vi "CheckExportedFunctionCallCoverage.vi"() -> ()   [LabVIEW 2020]
uses:
  <vilib>/Utility/traverseref.llb/TRef TravTarget.ctl
  02b7a759-a23e-437a-9814-93bb2d072b00.vi
  <vilib>/Utility/traverseref.llb/VI Scripting - Traverse.lvlib
panel:
  out "In Source but not called by LabVIEW":set{string}(c389)
  out "Specified in C++ Source":set{string}(c389)
  out "Called in LabIVEW":set{string}(c389)
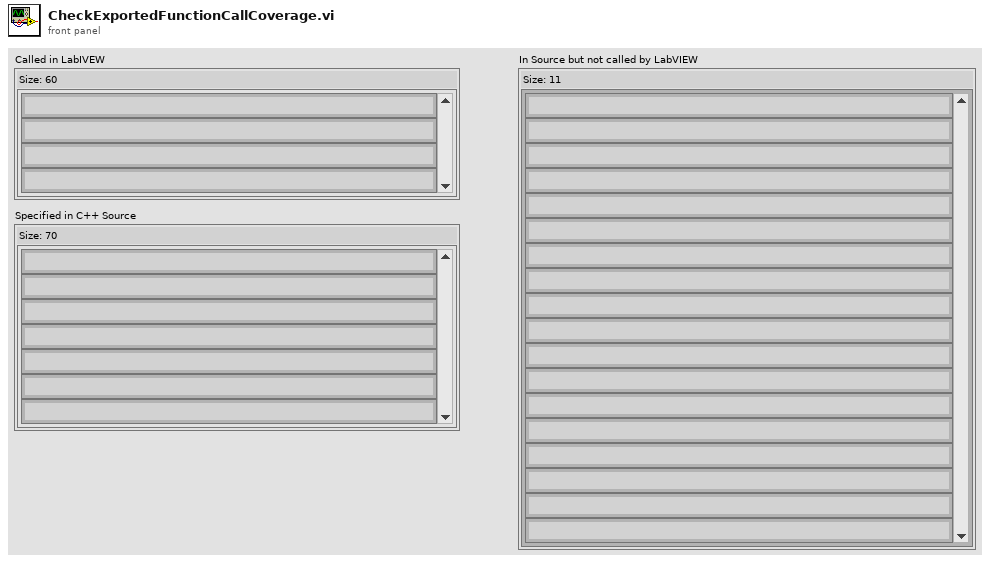
[diagram p1: front panel]
types:
  T1 = typedef "TRef TravTarget.ctl" = enum16{"FP", "BD", "Other"}
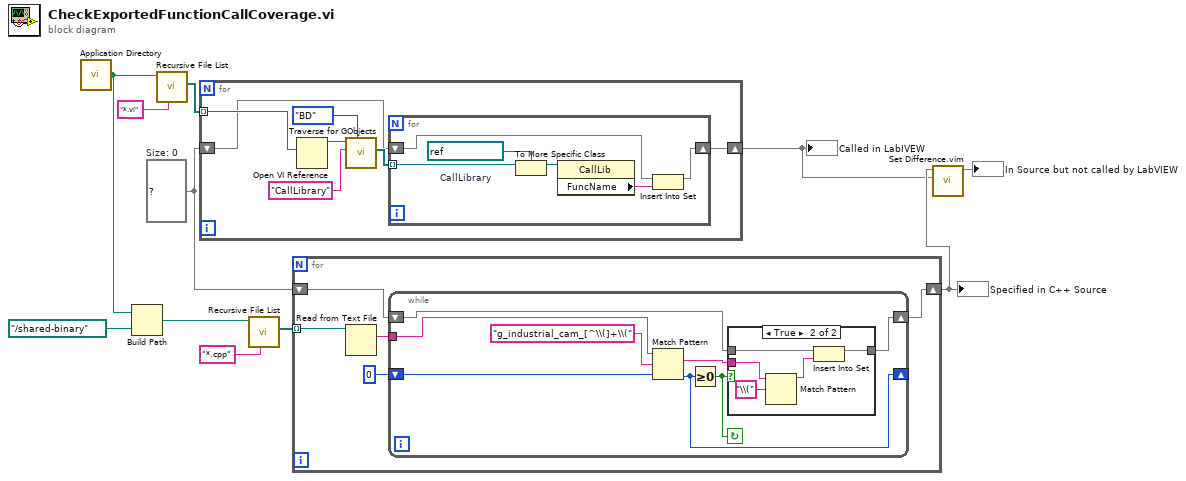
[diagram p0: block diagram]
diagram:
  w4 = set{string} {}  # Size: 0
  n1 = call <vilib>:"Application Directory.vi"() -> ("Application Directory"=w8:path)
  n2 = Build Path(base path=w8, name or relative path=path "../shared-binary") -> (appended path=w9:path)
  n3 = call <vilib>:"Recursive File List.vi"("pattern"="*.vi", "Folder Path"=w8) -> ("All Files in Dir"=w10:path[])  [unwired: 5 in, 4 out]
  n4 = for {
    tunnel: w10 -> [w18] mode=indexing
    shift-right: [w13] -> w2
    shift-left: w4 -> [w12]
    n5 = Open VI Reference(vi path=w18) -> (vi reference=w15:refnum<vi>)  [unwired: 5 in, 1 out]
    n6 = call <vilib>:"Traverse for GObjects.vi"("Traverse Target"=TRef_TravTarget."BD", "Class Name"="CallLibrary", "VI Refnum"=w15) -> ("References"=w16:refnum<vi>[])  [unwired: 5 in, 3 out]
    n7 = for {
      tunnel: w16 -> [w23] mode=indexing
      shift-right: [w20] -> w13
      shift-left: w12 -> [w19]
      w24 = refnum<vi> refnum  # CallLibrary
      n8 = To More Specific Class(target class=w24, reference=w23) -> (specific class reference=w22:refnum<vi>)  [unwired: 1 in, 1 out]
      n9 = property class="CallLib"(reference=w22) -> ("FuncName"=w21:string)  [unwired: 1 in, 2 out]
      n10 = Insert Into Set(10:w21, 11:w19) -> (3:w20:set{string})  [unwired: 1 out]
    }
  }
  "Called in LabIVEW" <- w2
  n11 = call <vilib>:"Recursive File List.vi"("pattern"="*.cpp", "Folder Path"=w9) -> ("All Files in Dir"=w5:path[])  [unwired: 5 in, 4 out]
  n12 = for {
    tunnel: w5 -> [w29] mode=indexing
    shift-right: [w26] -> w3
    shift-left: w4 -> [w27]
    n13 = Read from Text File(file (use dialog)=w29) -> (text=w25:string)  [unwired: 3 in, 3 out]
    n14 = while {
      shift-right: [w35] -> _
      shift-left: 0 ("offset (0)") -> [w36]
      shift-right: [w33] -> w26
      shift-left: w27 -> [w34]
      tunnel: w25 -> [w30]
      stop <- w31 continue-if-true
      n15 = Match Pattern(string=w30, regular expression="g_industrial_cam_[^\\(]+\\(", offset (0)=w36) -> (match substring=w32:string, offset past match=w35:i32)  [unwired: 2 out]
      n16 = Greater Or Equal To 0?(x=w35) -> (x >= 0?=w31:bool)
      n17 = case shown="True" w31 {
        tunnel: w34 -> [w38 w43]
        tunnel: [w38 w42] -> w33
        tunnel: w32 -> [_ w41]
        frame False {
        }
        frame True {
          n18 = Match Pattern(string=w41, regular expression="\\(") -> (before substring=w40:string)  [unwired: 1 in, 3 out]
          n19 = Insert Into Set(10:w40, 11:w43) -> (3:w42:set{string})  [unwired: 1 out]
        }
      }
    }
  }
  "Specified in C++ Source" <- w3
  n20 = call "Set Difference.vim"("set 2"=w2, "set 1"=w3) -> ("difference"=→"In Source but not called by LabVIEW":set{string})  [unwired: 9 in]
